vi "Begin.vi"(8 "error in":errorcluster) -> (0 "error out":errorcluster)   [LabVIEW 2020]
doc: "Called before other user functions, this VI can be used to open I/O refnums, load in file data, and do general program initialization. Notice that the <B>error out</B> terminal is simply used for data flow. Wiring it to other structures or subVIs ensures that this VI runs first."
uses:
  Robot Global Data.vi
  <vilib>/Rock Robotics/WPI/DriverStation/WPI_DriverStationRobotMode2.ctl
  <vilib>/Rock Robotics/WPI/Joystick/WPI_JoystickDeviceEnum.ctl
  <vilib>/Rock Robotics/WPI/RobotDrive/WPI_RobotDriveOpen2MotorWithExistingMotors.vi
  <vilib>/Rock Robotics/WPI/MotorControl/WPI_MotorControlOpen SPARK.vi
  <vilib>/Rock Robotics/SystemInterfaces/DIO/FPGA_DIOPWMChannel.ctl
  <vilib>/Rock Robotics/WPI/SafetyOutput/WPI_SafetyOutputConfigMenu.ctl
  <vilib>/Rock Robotics/WPI/Solenoid/WPI_SolenoidSetEnum.vi
  <vilib>/Rock Robotics/WPI/Solenoid/WPI_SolenoidChannel.ctl
  <vilib>/Rock Robotics/WPI/Solenoid/WPI_SolenoidValue.ctl
  <vilib>/Rock Robotics/Network Tables/NT Write Boolean Array.vi
  <vilib>/Rock Robotics/Network Tables/NT Write Numeric Array.vi
  <vilib>/Rock Robotics/WPI/Solenoid/WPI_SolenoidOpenDouble.vi
  <vilib>/Rock Robotics/SystemInterfaces/i2clib/i2c_bus.ctl
  <vilib>/Rock Robotics/Network Tables/NT Write Number.vi
panel:
  in  "Blue Calibration":cluster{"R":dbl, "G":dbl, "B":dbl}={"R"=0.143, "G"=0.427, "B"=0.429}
  in  "Green Calibration":cluster{"R":dbl, "G":dbl, "B":dbl}={"R"=0.197, "G"=0.561, "B"=0.24}
  in  "Red Calibration":cluster{"R":dbl, "G":dbl, "B":dbl}={"R"=0.561, "G"=0.323, "B"=0.114}
  in  "Yellow Calibration":cluster{"R":dbl, "G":dbl, "B":dbl}={"R"=0.361, "G"=0.524, "B"=0.113}
  in  "Calibration Time (sec)":u32=4
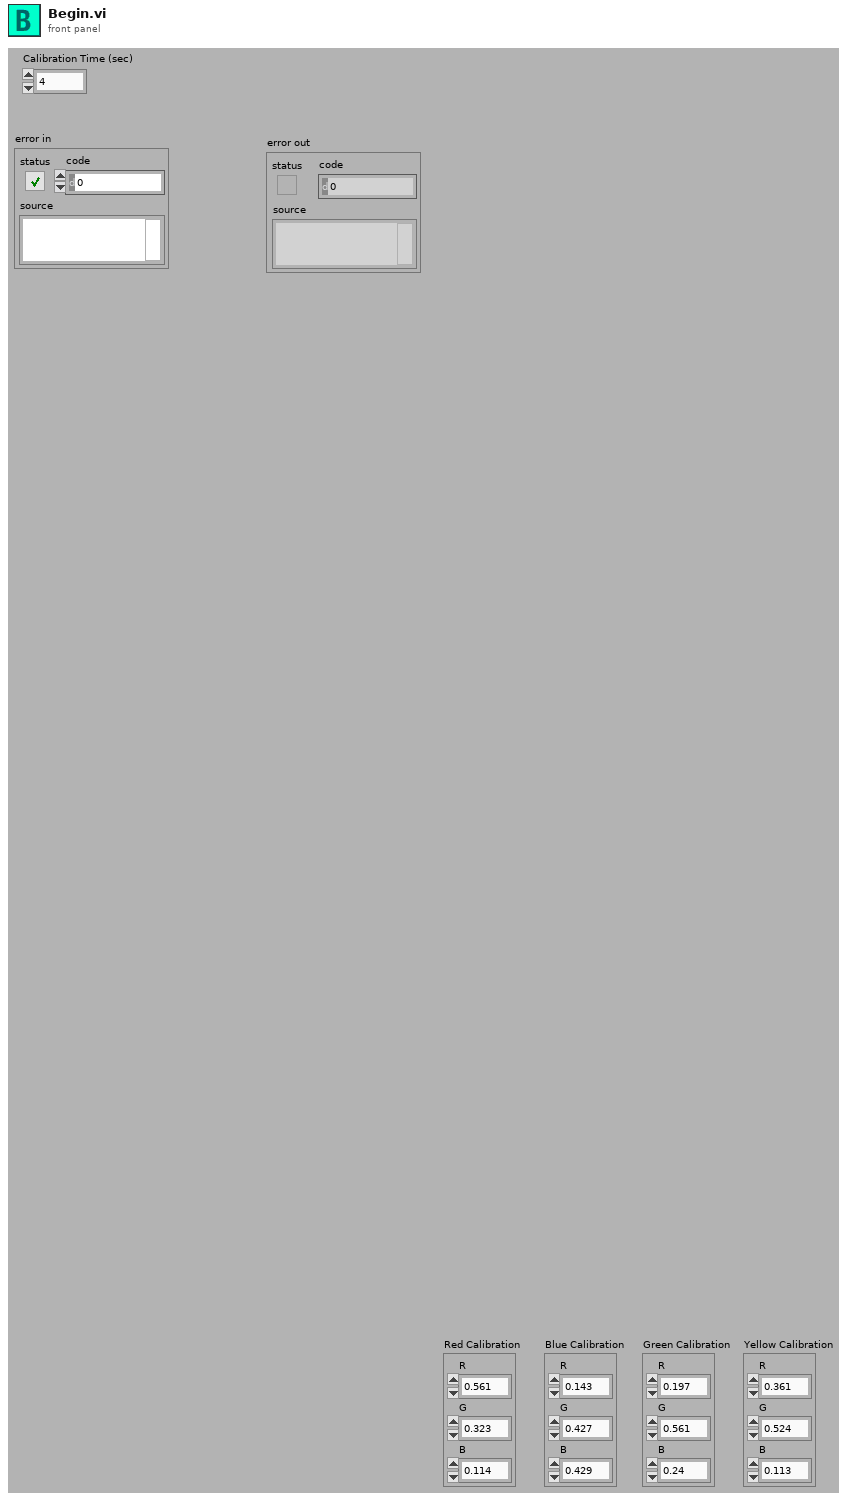
[diagram p1: front panel]
types:
  T1 = typedef "WPI_SolenoidChannel.ctl" = enum8{"Solenoid 0", "Solenoid 1", "Solenoid 2", "Solenoid 3", "Solenoid 4", "Solenoid 5", "Solenoid 6", "Solenoid 7", "Solenoid 8", "Solenoid 9", "Solenoid 10", "Solenoid 11", "Solenoid 12", "Solenoid 13", "Solenoid 14", "Solenoid 15", "Invalid"}
  T2 = typedef "WPI_SolenoidValue.ctl" = enum16{"Off", "On", "Forward", "Reverse"}
  T3 = typedef "WPI_SafetyOutputConfigMenu.ctl" = enum16{"Enable", "Disable"}
  T4 = typedef "i2c_bus.ctl" = enum16{"I2C On-Board", "I2C MXP", "Invalid"}
  T5 = typedef "FPGA_DIOPWMChannel.ctl" = enum8{"PWM 0", "PWM 1", "PWM 2", "PWM 3", "PWM 4", "PWM 5", "PWM 6", "PWM 7", "PWM 8", "PWM 9", "PWM MXP 0", "PWM MXP 1", "PWM MXP 2", "PWM MXP 3", "PWM MXP 4", "PWM MXP 5", "PWM MXP 6", "PWM MXP 7", "PWM MXP 8", "PWM MXP 9", "Invalid"}
  T6 = typedef "WPI_JoystickDeviceEnum.ctl" = enum16{"USB 0", "USB 1", "USB 2", "USB 3", "USB 4", "USB 5"}
  T7 = typedef "WPI_DriverStationRobotMode2.ctl" = enum16{"Autonomous Disabled", "Autonomous Enabled", "Teleop Disabled", "Teleop Enabled", "Disconnected", "Finish", "Test Disabled", "Test Enabled", "Emergency Stopped"}
  T8 = typedef "WPI_JoystickDevRef.ctl" = cluster{"Device":T6}
  T9 = typedef "WPI_MotorControlDeviceRef.ctl" = cluster{"DeviceStatus":errorcluster, "Type":T10, "PWM":cluster{"PWM Channel":T5, "DeadBand":T11}, "CAN":cluster{"Device Number":u8, "SetOutput VI Ref":variant, "GetOutput VI Ref":variant, "Enable VI Ref":variant, "Disable VI Ref":variant, "Data":variant}, "Invert":bool, "DIO PWM":cluster{"PWM \"Enable\" Channel":T5, "DIOChannel":T12, "PWM Rate":dbl}}
  T10 = typedef "WPI_MotorControlType.ctl" = enum16{"PWM", "CAN", "DIO PWM"}
  T11 = typedef "WPI_PWMDeadband.ctl" = cluster{"Name":string, "maxPositivePwm":i32, "minPositivePwm":i32, "centerPwm":i32, "maxNegativePwm":i32, "minNegativePwm":i32, "angularRange":u16}
  T12 = typedef "FPGA_DIOChannel.ctl" = enum8{"DIO 0", "DIO 1", "DIO 2", "DIO 3", "DIO 4", "DIO 5", "DIO 6", "DIO 7", "DIO 8", "DIO 9", "DIO MXP 0", "DIO MXP 1", "DIO MXP 2", "DIO MXP 3", "DIO MXP 4", "DIO MXP 5", "DIO MXP 6", "DIO MXP 7", "DIO MXP 8", "DIO MXP 9", "DIO MXP 10", "DIO MXP 11", "DIO MXP 12", "DIO MXP 13", "DIO MXP 14", "DIO MXP 15", "SPI Port CS1", "SPI Port CS2", "SPI Port CS3", "SPI Port MISO", "SPI Port MOSI", "Invalid"}
  T13 = typedef "WPI_RobotDriveDevRef.ctl" = cluster{"DevStatus":errorcluster, "Motors[]":T9[], "Square Inputs":bool, "Max Output":dbl}
  T14 = typedef "Color Sensor V3 DevRef.ctl" = cluster{"I2CDevRef":T15}
  T15 = typedef "WPI_I2CDevRef.ctl" = cluster{"DevStatus":errorcluster, "Device Address":u8, "Handle":i32, "I2C Bus":T4}
  T16 = typedef "WPI_SolenoidDevRef.ctl" = cluster{"DevStatus":errorcluster, "Pneumatics Control Module":u8, "Forward Solenoid Channel":T1, "Reverse Solenoid Channel":T1}
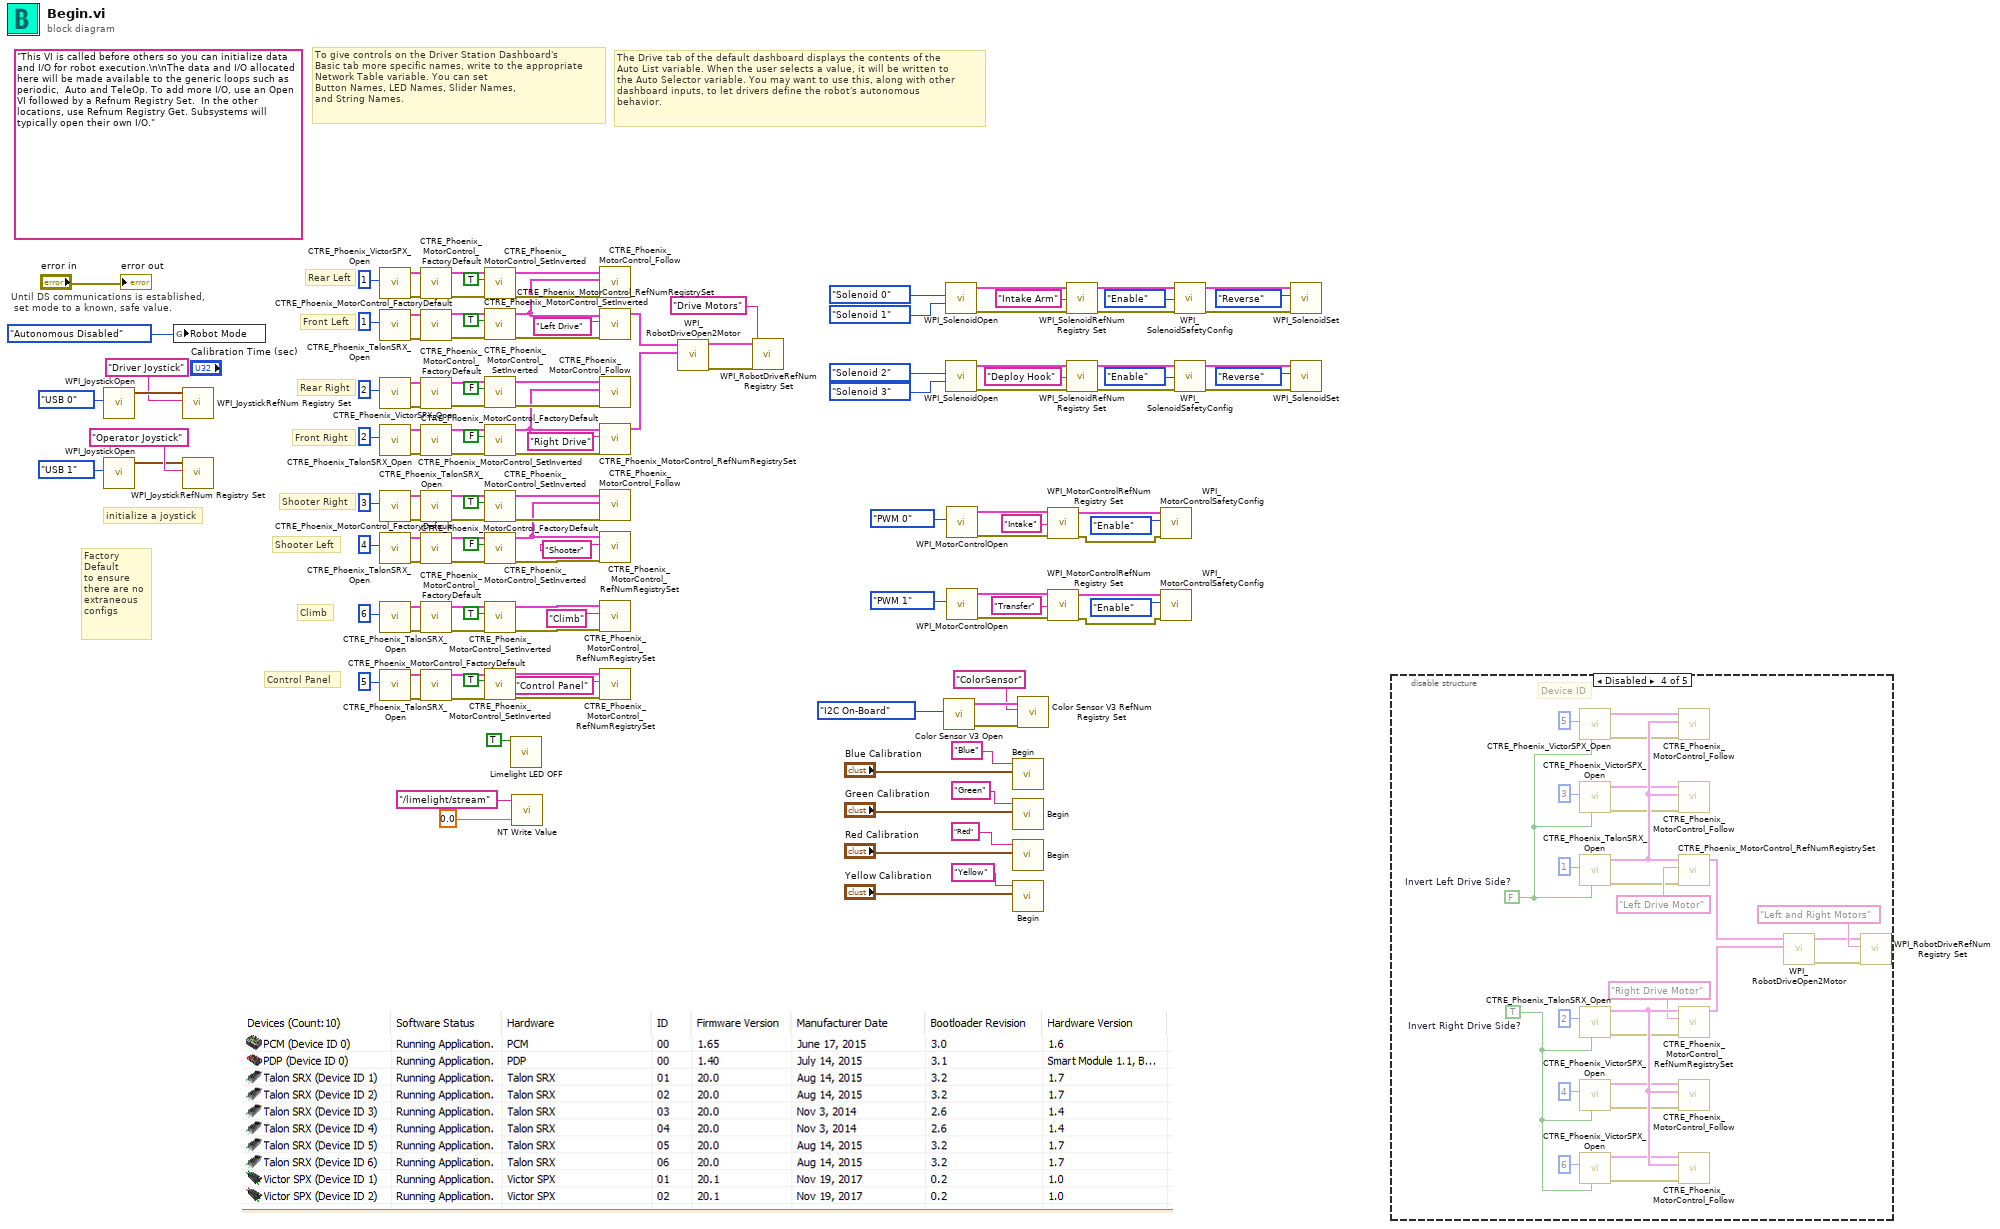
[diagram p0: block diagram]
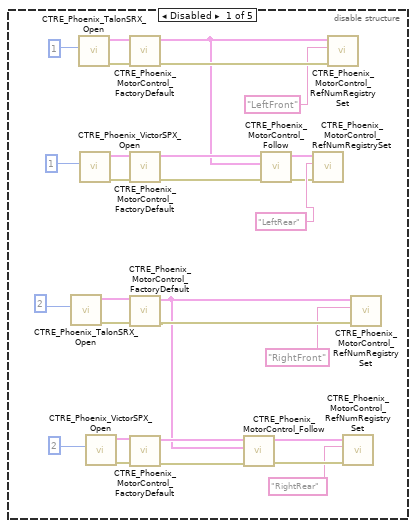
[diagram p2: hidden frame]
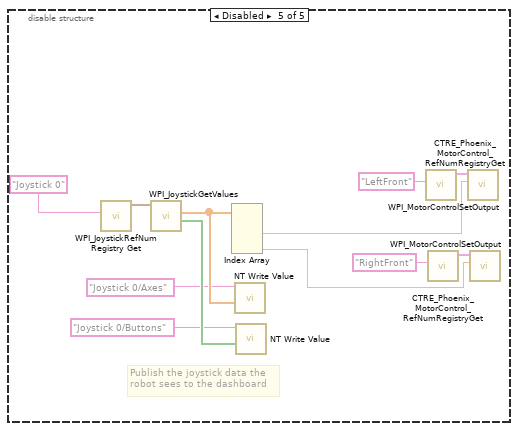
[diagram p5: hidden frame]
diagram:
  (unwired) "This VI is called before others so you can initialize data and I/O for robot execution.\n\nThe data and I/O allocated here will be made available to the generic loops such as periodic,  Auto and TeleOp. To add more I/O, use an Open VI followed by a Refnum Registry Set.  In the other locations, use Refnum Registry Get. Subsystems will typically open their own I/O."
  # "Climb"
  # "Control Panel"
  # "The Drive tab of the default dashboard displays the contents of the\nAuto List variable. When the user selects a value, it will be written to\nthe Auto Selector variable. You may want to use this, along with other\ndashboard inputs, to let drivers define the robot's autonomous\nbehavior."
  # "To give controls on the Driver Station Dashboard's\nBasic tab more specific names, write to the appropriate\nNetwork Table variable. You can set\nButton Names, LED Names, Slider Names,\nand String Names."
  # "Shooter Left"
  # "Shooter Right"
  # "Factory \nDefault \nto ensure \nthere are no \nextraneous \nconfigs"
  # "Front Right"
  # "Front Left"
  # "Rear Right"
  # "Rear Left"
  # "initialize a joystick"
  # "Until DS communications is established,\n set mode to a known, safe value."
  n1 = call <vilib>:"WPI_JoystickOpen.vi"("JoystickDevice"=WPI_JoystickDeviceEnum."USB 0") -> ("JoystickDevRef"=w116:T8)  [unwired: 10 in]
  n2 = call <vilib>:"WPI_JoystickOpen.vi"("JoystickDevice"=WPI_JoystickDeviceEnum."USB 1") -> ("JoystickDevRef"=w131:T8)  [unwired: 10 in]
  n3 = global write "Robot Global Data.vi" "Robot Mode"(WPI_DriverStationRobotMode2."Autonomous Disabled" ("Robot Mode")) -> ()
  n4 = call <vilib>:"WPI_JoystickRefNum Registry Set.vi"("refnum name"="Driver Joystick", "JoystickDevRef"=w116) -> ()  [unwired: 8 in, 2 out]
  n5 = call <vilib>:"WPI_JoystickRefNum Registry Set.vi"("refnum name"="Operator Joystick", "JoystickDevRef"=w131) -> ()  [unwired: 8 in, 2 out]
  n6 = call <vilib>:"CTRE_Phoenix_VictorSPX_Open.vi"("Device Number"=u8 1) -> ("error out"=w114:errorcluster, "PhoenixMotorControlDevRef"=w113:T9)  [unwired: 9 in]
  n7 = call <vilib>:"CTRE_Phoenix_TalonSRX_Open.vi"("Device Number"=u8 1) -> ("error out"=w111:errorcluster, "PhoenixMotorControlDevRef"=w112:T9)  [unwired: 9 in]
  n8 = call <vilib>:"CTRE_Phoenix_VictorSPX_Open.vi"("Device Number"=u8 2) -> ("error out"=w110:errorcluster, "PhoenixMotorControlDevRef"=w109:T9)  [unwired: 9 in]
  n9 = call <vilib>:"CTRE_Phoenix_TalonSRX_Open.vi"("Device Number"=u8 2) -> ("error out"=w108:errorcluster, "PhoenixMotorControlDevRef"=w107:T9)  [unwired: 9 in]
  n10 = call <vilib>:"CTRE_Phoenix_TalonSRX_Open.vi"("Device Number"=u8 3) -> ("error out"=w69:errorcluster, "PhoenixMotorControlDevRef"=w68:T9)  [unwired: 9 in]
  n11 = call <vilib>:"CTRE_Phoenix_TalonSRX_Open.vi"("Device Number"=u8 4) -> ("error out"=w67:errorcluster, "PhoenixMotorControlDevRef"=w66:T9)  [unwired: 9 in]
  n12 = call <vilib>:"CTRE_Phoenix_TalonSRX_Open.vi"("Device Number"=u8 6) -> ("error out"=w8:errorcluster, "PhoenixMotorControlDevRef"=w7:T9)  [unwired: 9 in]
  n13 = call <vilib>:"CTRE_Phoenix_TalonSRX_Open.vi"("Device Number"=u8 5) -> ("error out"=w42:errorcluster, "PhoenixMotorControlDevRef"=w41:T9)  [unwired: 9 in]
  n14 = call <vilib>:"CTRE_Phoenix_MotorControl_FactoryDefault.vi"("error in"=w114, "PhoenixMotorControlDevRef"=w113) -> ("error out"=w105:errorcluster, "PhoenixMotorControlDevRef"=w104:T9)  [unwired: 8 in]
  n15 = call <vilib>:"CTRE_Phoenix_MotorControl_FactoryDefault.vi"("error in"=w111, "PhoenixMotorControlDevRef"=w112) -> ("error out"=w99:errorcluster, "PhoenixMotorControlDevRef"=w100:T9)  [unwired: 8 in]
  n16 = call <vilib>:"CTRE_Phoenix_MotorControl_FactoryDefault.vi"("error in"=w110, "PhoenixMotorControlDevRef"=w109) -> ("error out"=w95:errorcluster, "PhoenixMotorControlDevRef"=w94:T9)  [unwired: 8 in]
  n17 = call <vilib>:"CTRE_Phoenix_MotorControl_FactoryDefault.vi"("error in"=w108, "PhoenixMotorControlDevRef"=w107) -> ("error out"=w90:errorcluster, "PhoenixMotorControlDevRef"=w89:T9)  [unwired: 8 in]
  n18 = call <vilib>:"CTRE_Phoenix_MotorControl_FactoryDefault.vi"("error in"=w69, "PhoenixMotorControlDevRef"=w68) -> ("error out"=w63:errorcluster, "PhoenixMotorControlDevRef"=w64:T9)  [unwired: 8 in]
  n19 = call <vilib>:"CTRE_Phoenix_MotorControl_FactoryDefault.vi"("error in"=w67, "PhoenixMotorControlDevRef"=w66) -> ("error out"=w58:errorcluster, "PhoenixMotorControlDevRef"=w59:T9)  [unwired: 8 in]
  n20 = call <vilib>:"CTRE_Phoenix_MotorControl_FactoryDefault.vi"("error in"=w8, "PhoenixMotorControlDevRef"=w7) -> ("error out"=w4:errorcluster, "PhoenixMotorControlDevRef"=w5:T9)  [unwired: 8 in]
  n21 = call <vilib>:"CTRE_Phoenix_MotorControl_FactoryDefault.vi"("error in"=w42, "PhoenixMotorControlDevRef"=w41) -> ("error out"=w38:errorcluster, "PhoenixMotorControlDevRef"=w39:T9)  [unwired: 8 in]
  n22 = call <vilib>:"CTRE_Phoenix_MotorControl_SetInverted.vi"("error in (no error)"=w105, "Invert?"=TRUE, "PhoenixMotorControlDevRef"=w104) -> ("error out"=w102:errorcluster, "PhoenixMotorControlDevRef"=w103:T9)  [unwired: 7 in]
  n23 = call <vilib>:"CTRE_Phoenix_MotorControl_SetInverted.vi"("error in (no error)"=w99, "Invert?"=TRUE, "PhoenixMotorControlDevRef"=w100) -> ("error out"=w98:errorcluster, "PhoenixMotorControlDevRef"=w97:T9)  [unwired: 7 in]
  n24 = call <vilib>:"CTRE_Phoenix_MotorControl_SetInverted.vi"("error in (no error)"=w95, "Invert?"=FALSE, "PhoenixMotorControlDevRef"=w94) -> ("error out"=w92:errorcluster, "PhoenixMotorControlDevRef"=w93:T9)  [unwired: 7 in]
  n25 = call <vilib>:"CTRE_Phoenix_MotorControl_SetInverted.vi"("error in (no error)"=w90, "Invert?"=FALSE, "PhoenixMotorControlDevRef"=w89) -> ("error out"=w87:errorcluster, "PhoenixMotorControlDevRef"=w88:T9)  [unwired: 7 in]
  n26 = call <vilib>:"CTRE_Phoenix_MotorControl_SetInverted.vi"("error in (no error)"=w63, "Invert?"=TRUE, "PhoenixMotorControlDevRef"=w64) -> ("error out"=w62:errorcluster, "PhoenixMotorControlDevRef"=w61:T9)  [unwired: 7 in]
  n27 = call <vilib>:"CTRE_Phoenix_MotorControl_SetInverted.vi"("error in (no error)"=w58, "Invert?"=FALSE, "PhoenixMotorControlDevRef"=w59) -> ("error out"=w57:errorcluster, "PhoenixMotorControlDevRef"=w56:T9)  [unwired: 7 in]
  n28 = call <vilib>:"CTRE_Phoenix_MotorControl_SetInverted.vi"("error in (no error)"=w4, "Invert?"=TRUE, "PhoenixMotorControlDevRef"=w5) -> ("error out"=w3:errorcluster, "PhoenixMotorControlDevRef"=w2:T9)  [unwired: 7 in]
  n29 = call <vilib>:"CTRE_Phoenix_MotorControl_SetInverted.vi"("error in (no error)"=w38, "Invert?"=TRUE, "PhoenixMotorControlDevRef"=w39) -> ("error out"=w37:errorcluster, "PhoenixMotorControlDevRef"=w36:T9)  [unwired: 7 in]
  n30 = call "Limelight LED OFF.vi"("D Select  8"=TRUE) -> ()  [unwired: 11 in]
  n31 = call-poly <vilib>:"NT Write Value.vi"("Numeric"=0.0, "Name"="/limelight/stream") -> ()  [unwired: 9 in, 1 out]
  n32 = call <vilib>:"CTRE_Phoenix_MotorControl_Follow.vi"("error in (no error)"=w102, "Master Controller to Follow"=w97, "PhoenixMotorControlDevRef"=w103) -> ()  [unwired: 7 in, 2 out]
  n33 = call <vilib>:"CTRE_Phoenix_MotorControl_RefNumRegistrySet.vi"("error in (no error)"=w98, "refnum name"="Left Drive", "PhoenixMotorControlDevRef"=w97) -> ("PhoenixMotorControlDevRef"=w124:T9)  [unwired: 7 in, 1 out]
  n34 = call <vilib>:"CTRE_Phoenix_MotorControl_Follow.vi"("error in (no error)"=w92, "Master Controller to Follow"=w88, "PhoenixMotorControlDevRef"=w93) -> ()  [unwired: 7 in, 2 out]
  n35 = call <vilib>:"CTRE_Phoenix_MotorControl_RefNumRegistrySet.vi"("error in (no error)"=w87, "refnum name"="Right Drive", "PhoenixMotorControlDevRef"=w88) -> ("PhoenixMotorControlDevRef"=w123:T9)  [unwired: 7 in, 1 out]
  n36 = call <vilib>:"CTRE_Phoenix_MotorControl_Follow.vi"("error in (no error)"=w62, "Master Controller to Follow"=w56, "PhoenixMotorControlDevRef"=w61) -> ()  [unwired: 7 in, 2 out]
  n37 = call <vilib>:"CTRE_Phoenix_MotorControl_RefNumRegistrySet.vi"("error in (no error)"=w57, "refnum name"="Shooter", "PhoenixMotorControlDevRef"=w56) -> ()  [unwired: 7 in, 2 out]
  n38 = call <vilib>:"CTRE_Phoenix_MotorControl_RefNumRegistrySet.vi"("error in (no error)"=w3, "refnum name"="Climb", "PhoenixMotorControlDevRef"=w2) -> ()  [unwired: 7 in, 2 out]
  n39 = call <vilib>:"CTRE_Phoenix_MotorControl_RefNumRegistrySet.vi"("error in (no error)"=w37, "refnum name"="Control Panel", "PhoenixMotorControlDevRef"=w36) -> ()  [unwired: 7 in, 2 out]
  n40 = call-poly <vilib>:"WPI_RobotDriveOpen2Motor.vi"("Right Motor Dev Ref"=w123, "Left Motor Dev Ref"=w124) -> ("error out"=w119:errorcluster, "RobotDriveDevRef"=w120:T13)  [unwired: 8 in]
  n41 = call <vilib>:"WPI_RobotDriveRefNum Registry Set.vi"("error in (no error)"=w119, "refnum name"="Drive Motors", "RobotDriveDevRef"=w120) -> ()  [unwired: 7 in, 2 out]
  n42 = call <vilib>:"Color Sensor V3 Open.vi"("I2C Bus"=i2c_bus."I2C On-Board") -> ("error out"=w33:errorcluster, "ColorSensorDevRef"=w34:T14)  [unwired: 9 in]
  n43 = call-poly <vilib>:"WPI_SolenoidOpen.vi"("Reverse Solenoid Channel"=WPI_SolenoidChannel."Solenoid 1" ("Solenoid Channel"), "Forward Solenoid Channel"=WPI_SolenoidChannel."Solenoid 0" ("Solenoid Channel")) -> ("error out"=w52:errorcluster, "SolenoidDevRef"=w55:T16)  [unwired: 8 in]
  n44 = call-poly <vilib>:"WPI_SolenoidOpen.vi"("Reverse Solenoid Channel"=WPI_SolenoidChannel."Solenoid 3" ("Solenoid Channel"), "Forward Solenoid Channel"=WPI_SolenoidChannel."Solenoid 2" ("Solenoid Channel")) -> ("error out"=w15:errorcluster, "SolenoidDevRef"=w12:T16)  [unwired: 8 in]
  n45 = call-poly <vilib>:"WPI_MotorControlOpen.vi"("PWM Channel"=FPGA_DIOPWMChannel."PWM 0") -> ("error out"=w81:errorcluster, "MotorControlDeviceRef"=w85:T9)  [unwired: 9 in]
  n46 = call-poly <vilib>:"WPI_MotorControlOpen.vi"("PWM Channel"=FPGA_DIOPWMChannel."PWM 1") -> ("error out"=w78:errorcluster, "MotorControlDeviceRef"=w74:T9)  [unwired: 9 in]
  n47 = call "Begin.vi"(10:"Blue Calibration", 11:"Blue" ("Name")) -> ()  [unwired: 9 in, 1 out]
  n48 = call "Begin.vi"(10:"Green Calibration", 11:"Green" ("Name")) -> ()  [unwired: 9 in, 1 out]
  n49 = call "Begin.vi"(10:"Red Calibration", 11:"Red" ("Name")) -> ()  [unwired: 9 in, 1 out]
  n50 = call "Begin.vi"(10:"Yellow Calibration", 11:"Yellow" ("Name")) -> ()  [unwired: 9 in, 1 out]
  n51 = call <vilib>:"Color Sensor V3 RefNum Registry Set.vi"("error in (no error)"=w33, "refnum name"="ColorSensor", "ColorSensorDevRef"=w34) -> ()  [unwired: 7 in, 2 out]
  n52 = call <vilib>:"WPI_MotorControlRefNum Registry Set.vi"("error in (no error)"=w81, "refnum name"="Intake", "MotorControlDevRef"=w85) -> ("error out"=w80:errorcluster, "MotorControlDevRef"=w84:T9)  [unwired: 7 in]
  n53 = call <vilib>:"WPI_MotorControlRefNum Registry Set.vi"("error in (no error)"=w78, "refnum name"="Transfer", "MotorControlDevRef"=w74) -> ("error out"=w79:errorcluster, "MotorControlDevRef"=w75:T9)  [unwired: 7 in]
  n54 = call <vilib>:"WPI_SolenoidRefNum Registry Set.vi"("error in (no error)"=w52, "refnum name"="Intake Arm", "SolenoidDevRef"=w55) -> ("error out"=w51:errorcluster, "SolenoidDevRef"=w54:T16)  [unwired: 7 in]
  n55 = call <vilib>:"WPI_SolenoidRefNum Registry Set.vi"("error in (no error)"=w15, "refnum name"="Deploy Hook", "SolenoidDevRef"=w12) -> ("error out"=w16:errorcluster, "SolenoidDevRef"=w13:T16)  [unwired: 7 in]
  n56 = call <vilib>:"WPI_MotorControlSafetyConfig.vi"("error in (no error)"=w80, "mode"=WPI_SafetyOutputConfigMenu."Enable", "MotorControlDevRef"=w84) -> ()  [unwired: 7 in, 2 out]
  n57 = call <vilib>:"WPI_MotorControlSafetyConfig.vi"("error in (no error)"=w79, "mode"=WPI_SafetyOutputConfigMenu."Enable", "MotorControlDevRef"=w75) -> ()  [unwired: 7 in, 2 out]
  n58 = call <vilib>:"WPI_SolenoidSafetyConfig.vi"("error in (no error)"=w51, "mode"=WPI_SafetyOutputConfigMenu."Enable", "SolenoidDevRef"=w54) -> ("error out"=w50:errorcluster, "SolenoidDevRef"=w53:T16)  [unwired: 7 in]
  n59 = call <vilib>:"WPI_SolenoidSafetyConfig.vi"("error in (no error)"=w16, "mode"=WPI_SafetyOutputConfigMenu."Enable", "SolenoidDevRef"=w13) -> ("error out"=w17:errorcluster, "SolenoidDevRef"=w14:T16)  [unwired: 7 in]
  n60 = call-poly <vilib>:"WPI_SolenoidSet.vi"("error in (no error)"=w50, "Value"=WPI_SolenoidValue."Reverse", "SolenoidDevRef"=w53) -> ()  [unwired: 7 in, 2 out]
  n61 = call-poly <vilib>:"WPI_SolenoidSet.vi"("error in (no error)"=w17, "Value"=WPI_SolenoidValue."Reverse", "SolenoidDevRef"=w14) -> ()  [unwired: 7 in, 2 out]
  n62 = disable-structure shown="Disabled" {
    frame Disabled {
      n63 = call <vilib>:"CTRE_Phoenix_TalonSRX_Open.vi"("Device Number"=u8 2) -> ("error out"=w158:errorcluster, "PhoenixMotorControlDevRef"=w148:T9)  [unwired: 9 in]
      n64 = call <vilib>:"CTRE_Phoenix_TalonSRX_Open.vi"("Device Number"=u8 1) -> ("error out"=w156:errorcluster, "PhoenixMotorControlDevRef"=w146:T9)  [unwired: 9 in]
      n65 = call <vilib>:"CTRE_Phoenix_VictorSPX_Open.vi"("Device Number"=u8 1) -> ("error out"=w154:errorcluster, "PhoenixMotorControlDevRef"=w152:T9)  [unwired: 9 in]
      n66 = call <vilib>:"CTRE_Phoenix_VictorSPX_Open.vi"("Device Number"=u8 2) -> ("error out"=w160:errorcluster, "PhoenixMotorControlDevRef"=w150:T9)  [unwired: 9 in]
      n67 = call <vilib>:"CTRE_Phoenix_MotorControl_FactoryDefault.vi"("error in"=w156, "PhoenixMotorControlDevRef"=w146) -> ("error out"=w157:errorcluster, "PhoenixMotorControlDevRef"=w147:T9)  [unwired: 8 in]
      n68 = call <vilib>:"CTRE_Phoenix_MotorControl_FactoryDefault.vi"("error in"=w154, "PhoenixMotorControlDevRef"=w152) -> ("error out"=w155:errorcluster, "PhoenixMotorControlDevRef"=w153:T9)  [unwired: 8 in]
      n69 = call <vilib>:"CTRE_Phoenix_MotorControl_FactoryDefault.vi"("error in"=w158, "PhoenixMotorControlDevRef"=w148) -> ("error out"=w159:errorcluster, "PhoenixMotorControlDevRef"=w149:T9)  [unwired: 8 in]
      n70 = call <vilib>:"CTRE_Phoenix_MotorControl_FactoryDefault.vi"("error in"=w160, "PhoenixMotorControlDevRef"=w150) -> ("error out"=w161:errorcluster, "PhoenixMotorControlDevRef"=w151:T9)  [unwired: 8 in]
      n71 = call <vilib>:"CTRE_Phoenix_MotorControl_Follow.vi"("error in (no error)"=w161, "Master Controller to Follow"=w149, "PhoenixMotorControlDevRef"=w151) -> ("error out"=w144:errorcluster, "PhoenixMotorControlDevRef"=w145:T9)  [unwired: 7 in]
      n72 = call <vilib>:"CTRE_Phoenix_MotorControl_Follow.vi"("error in (no error)"=w155, "Master Controller to Follow"=w147, "PhoenixMotorControlDevRef"=w153) -> ("error out"=w136:errorcluster, "PhoenixMotorControlDevRef"=w137:T9)  [unwired: 7 in]
      n73 = call <vilib>:"CTRE_Phoenix_MotorControl_RefNumRegistrySet.vi"("error in (no error)"=w136, "refnum name"="LeftRear", "PhoenixMotorControlDevRef"=w137) -> ()  [unwired: 7 in, 2 out]
      n74 = call <vilib>:"CTRE_Phoenix_MotorControl_RefNumRegistrySet.vi"("error in (no error)"=w157, "refnum name"="LeftFront", "PhoenixMotorControlDevRef"=w147) -> ()  [unwired: 7 in, 2 out]
      n75 = call <vilib>:"CTRE_Phoenix_MotorControl_RefNumRegistrySet.vi"("error in (no error)"=w144, "refnum name"="RightRear", "PhoenixMotorControlDevRef"=w145) -> ()  [unwired: 7 in, 2 out]
      n76 = call <vilib>:"CTRE_Phoenix_MotorControl_RefNumRegistrySet.vi"("error in (no error)"=w159, "refnum name"="RightFront", "PhoenixMotorControlDevRef"=w149) -> ()  [unwired: 7 in, 2 out]
    }
    frame Enabled {
    }
    frame Disabled {
    }
    frame Disabled {
      w188 = FALSE  # Invert Left Drive Side?
      w187 = TRUE  # Invert Right Drive Side?
      # "Device ID"
      n77 = call <vilib>:"CTRE_Phoenix_VictorSPX_Open.vi"("Invert"=w188, "Device Number"=u8 5) -> ("error out"=w178:errorcluster, "PhoenixMotorControlDevRef"=w179:T9)  [unwired: 8 in]
      n78 = call <vilib>:"CTRE_Phoenix_VictorSPX_Open.vi"("Invert"=w188, "Device Number"=u8 3) -> ("error out"=w177:errorcluster, "PhoenixMotorControlDevRef"=w180:T9)  [unwired: 8 in]
      n79 = call <vilib>:"CTRE_Phoenix_TalonSRX_Open.vi"("Invert"=w188, "Device Number"=u8 1) -> ("error out"=w168:errorcluster, "PhoenixMotorControlDevRef"=w181:T9)  [unwired: 8 in]
      n80 = call <vilib>:"CTRE_Phoenix_TalonSRX_Open.vi"("Invert"=w187, "Device Number"=u8 2) -> ("error out"=w169:errorcluster, "PhoenixMotorControlDevRef"=w176:T9)  [unwired: 8 in]
      n81 = call <vilib>:"CTRE_Phoenix_VictorSPX_Open.vi"("Invert"=w187, "Device Number"=u8 4) -> ("error out"=w172:errorcluster, "PhoenixMotorControlDevRef"=w173:T9)  [unwired: 8 in]
      n82 = call <vilib>:"CTRE_Phoenix_VictorSPX_Open.vi"("Invert"=w187, "Device Number"=u8 6) -> ("error out"=w175:errorcluster, "PhoenixMotorControlDevRef"=w174:T9)  [unwired: 8 in]
      n83 = call <vilib>:"CTRE_Phoenix_MotorControl_Follow.vi"("error in (no error)"=w178, "Master Controller to Follow"=w181, "PhoenixMotorControlDevRef"=w179) -> ()  [unwired: 7 in, 2 out]
      n84 = call <vilib>:"CTRE_Phoenix_MotorControl_Follow.vi"("error in (no error)"=w177, "Master Controller to Follow"=w181, "PhoenixMotorControlDevRef"=w180) -> ()  [unwired: 7 in, 2 out]
      n85 = call <vilib>:"CTRE_Phoenix_MotorControl_RefNumRegistrySet.vi"("error in (no error)"=w168, "refnum name"="Left Drive Motor", "PhoenixMotorControlDevRef"=w181) -> ("PhoenixMotorControlDevRef"=w182:T9)  [unwired: 7 in, 1 out]
      n86 = call <vilib>:"CTRE_Phoenix_MotorControl_RefNumRegistrySet.vi"("error in (no error)"=w169, "refnum name"="Right Drive Motor", "PhoenixMotorControlDevRef"=w176) -> ("PhoenixMotorControlDevRef"=w183:T9)  [unwired: 7 in, 1 out]
      n87 = call <vilib>:"CTRE_Phoenix_MotorControl_Follow.vi"("error in (no error)"=w172, "Master Controller to Follow"=w176, "PhoenixMotorControlDevRef"=w173) -> ()  [unwired: 7 in, 2 out]
      n88 = call <vilib>:"CTRE_Phoenix_MotorControl_Follow.vi"("error in (no error)"=w175, "Master Controller to Follow"=w176, "PhoenixMotorControlDevRef"=w174) -> ()  [unwired: 7 in, 2 out]
      n89 = call-poly <vilib>:"WPI_RobotDriveOpen2Motor.vi"("Right Motor Dev Ref"=w183, "Left Motor Dev Ref"=w182) -> ("error out"=w184:errorcluster, "RobotDriveDevRef"=w185:T13)  [unwired: 8 in]
      n90 = call <vilib>:"WPI_RobotDriveRefNum Registry Set.vi"("error in (no error)"=w184, "refnum name"="Left and Right Motors", "RobotDriveDevRef"=w185) -> ()  [unwired: 7 in, 2 out]
    }
    frame Disabled {
      # "Publish the joystick data the\nrobot sees to the dashboard"
      n91 = call <vilib>:"WPI_JoystickRefNum Registry Get.vi"("refnum name"="Joystick 0") -> ("JoystickDevRef"=w190:T8)  [unwired: 1 in, 9 out]
      n92 = call <vilib>:"WPI_JoystickGetValues.vi"("JoystickDevRef"=w190) -> ("Buttons"=w194:bool[], "Axes"=w193:dbl[])  [unwired: 6 in, 3 out]
      n93 = Index Array(array=w193) -> (element #2=w197:dbl, element #4=w200:dbl)  [unwired: 4 in, 2 out]
      n94 = call-poly <vilib>:"NT Write Value.vi"("Numeric Array"=w193, "Name"="Joystick 0/Axes") -> ()  [unwired: 9 in, 1 out]
      n95 = call-poly <vilib>:"NT Write Value.vi"("Boolean Array"=w194, "Name"="Joystick 0/Buttons") -> ()  [unwired: 9 in, 1 out]
      n96 = call <vilib>:"CTRE_Phoenix_MotorControl_RefNumRegistryGet.vi"("refnum name"="LeftFront") -> ("PhoenixMotorControlDevRef"=w196:T9)  [unwired: 9 in, 1 out]
      n97 = call <vilib>:"CTRE_Phoenix_MotorControl_RefNumRegistryGet.vi"("refnum name"="RightFront") -> ("PhoenixMotorControlDevRef"=w199:T9)  [unwired: 9 in, 1 out]
      n98 = call <vilib>:"WPI_MotorControlSetOutput.vi"("Output"=w197, "MotorControlDevRef"=w196) -> ()  [unwired: 7 in, 3 out]
      n99 = call <vilib>:"WPI_MotorControlSetOutput.vi"("Output"=w200, "MotorControlDevRef"=w199) -> ()  [unwired: 7 in, 3 out]
    }
  }
  "error out" <- "error in"
